vi "Run Optimization.vi"(8 "error in":errorcluster, 11 "Generic Optimization":refnum<class "Generic Optimization.lvclass">) -> (0 "error out":errorcluster, 3 "Generic Optimization out":refnum<class "Generic Optimization.lvclass">)   [LabVIEW 2018, in "Generic Optimization Actor.lvlib" / "Generic Optimization.lvclass"]
uses:
  Generic Optimization.lvclass
  C:/Users/Administrator/Desktop/LabVIEW EMS/EMS Generic Actor/EMS Generic/EMS Generic.lvclass
  Generic Optimization.lvclass/Generic Optimization.ctl
  EMS Generic Actor/EMS Generic/EMS Generic.lvclass
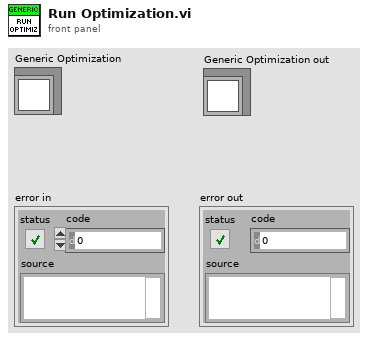
[diagram p1: front panel]
types:
  T1 = typedef "Generic Optimization Actor.lvlib/Generic Optimization.lvclass/Optimization Results Cluster.ctl" = cluster{"negated_net_battery_hold":dbl[][], " reactive_hold":dbl[][], " generatorpower_hold":dbl[][], " generatorreactive_hold":dbl[][], " PV_hold":dbl[][], "PCC_hold[0]":dbl[], " QCC_hold[0]":dbl[], " ES_VF_Controller":dbl[], " GEN_VF_Controller":dbl[], " voltage_hold":dbl[][], " SOC_hold":dbl[][], " Status":string}
  T2 = typedef "Generic Optimization Actor.lvlib/Generic Optimization.lvclass/Optimization Data Cluster.ctl" = cluster{"ES_BUS_ID":dbl[], "ES_VF_Controller":dbl[], "ES_Measurement_SOC":dbl[], "ES_Power_Rating":dbl[], "ES_Energy_Rating":dbl[], "ES_PowerFactor":dbl[], "ES_ChargeEffic":dbl[], "ES_DischargeEffic":dbl[], "ES_min_SOC":dbl[], "ES_max_SOC":dbl[], "GEN_BUS_ID":dbl[], "GEN_VF_Controller":dbl[], "GEN_Min_Power":dbl[], "GEN_Power_Rating":dbl[], "GEN_MaxPF_Lead":dbl[], "GEN_MaxPF_Lag":dbl[], "GEN_Marginal_Cost":dbl[][], "GEN_Marginal_Power":dbl[][], "GEN_Start_Cost":dbl[], "LOAD_BUS_ID":dbl[], "ForecastDataLongLoadP":dbl[][], "ForecastDataLongLoadQ":dbl[][], "PV_BUS_ID":dbl[], "PV_PowerRating_kVA":dbl[], "ForecastDataLongPV":dbl[][], "RealTimePrice":dbl[], "Forecast_dt":dbl, "Bus_Number":dbl[], "Bus_Voltage_Min":dbl[], "Bus_Voltage_Max":dbl[], "Bus_Voltage_Measured":dbl[], "Bus_Voltage_Nominal":dbl[], "From_Bus":dbl[], "To_Bus":dbl[], "Network_resistance":dbl[], "Network_reactance":dbl[], "Power_Flow_Limit":dbl[][], "Linear_PieceWise_PowerFLow":dbl[][], "Reactive_Flow_Limit":dbl[][], "Linear_PieceWise_ReactiveFLow":dbl[][], "PCC_min":dbl[], "PCC_max":dbl[], "QCC_min":dbl[], "QCC_max":dbl[], "Optimization_Type":i32, "Grid_State":i32}
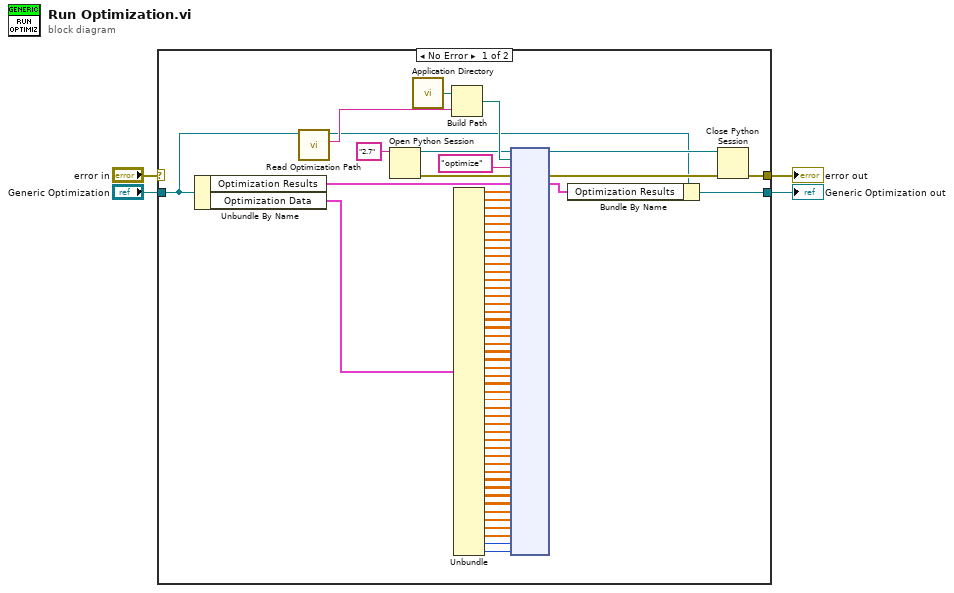
[diagram p0: block diagram]
diagram:
  n1 = case shown="No Error" "error in" {
    selector: "error in" -> [_ w68]
    tunnel: [w8 w68] -> w4
    tunnel: "Generic Optimization" -> [w7 w67]
    tunnel: [w14 w67] -> w1
    frame No Error {
      n2 = Unbundle By Name(w7) -> ("Optimization Results"=w63:T1, "Optimization Data"=w62:T2)
      n3 = call "Read Optimization Path.vi"("EMS Generic in"=w7) -> ("Optimization Relative Path"=w6:string, "EMS Generic out"=w5:refnum<class "Generic Optimization.lvclass">)  [unwired: 8 in, 1 out]
      n4 = Open Python Session(python version="2.7" ("Python version")) -> (session out=w12:refnum<k35>, error out=w11:errorcluster)  [unwired: 2 in]
      n5 = call <vilib>:"Application Directory.vi"() -> ("Application Directory"=w65:path)
      n6 = Build Path(base path=w65, name or relative path=w6) -> (appended path=w64:path)
      n7 = Unbundle(w62) -> ("ES_BUS_ID"=w61:dbl[], "ES_VF_Controller"=w60:dbl[], "ES_Measurement_SOC"=w59:dbl[], "ES_Power_Rating"=w58:dbl[], "ES_Energy_Rating"=w57:dbl[], "ES_PowerFactor"=w56:dbl[], "ES_ChargeEffic"=w55:dbl[], "ES_DischargeEffic"=w54:dbl[], "ES_min_SOC"=w53:dbl[], "ES_max_SOC"=w52:dbl[], "GEN_BUS_ID"=w51:dbl[], "GEN_VF_Controller"=w50:dbl[], "GEN_Min_Power"=w49:dbl[], "GEN_Power_Rating"=w48:dbl[], "GEN_MaxPF_Lead"=w47:dbl[], "GEN_MaxPF_Lag"=w46:dbl[], "GEN_Marginal_Cost"=w45:dbl[][], "GEN_Marginal_Power"=w44:dbl[][], "GEN_Start_Cost"=w43:dbl[], "LOAD_BUS_ID"=w42:dbl[], "ForecastDataLongLoadP"=w41:dbl[][], "ForecastDataLongLoadQ"=w40:dbl[][], "PV_BUS_ID"=w39:dbl[], "PV_PowerRating_kVA"=w38:dbl[], "ForecastDataLongPV"=w37:dbl[][], "RealTimePrice"=w36:dbl[], "Forecast_dt"=w35:dbl, "Bus_Number"=w34:dbl[], "Bus_Voltage_Min"=w33:dbl[], "Bus_Voltage_Max"=w32:dbl[], "Bus_Voltage_Measured"=w31:dbl[], "Bus_Voltage_Nominal"=w30:dbl[], "From_Bus"=w29:dbl[], "To_Bus"=w28:dbl[], "Network_resistance"=w27:dbl[], "Network_reactance"=w26:dbl[], "Power_Flow_Limit"=w25:dbl[][], "Linear_PieceWise_PowerFLow"=w24:dbl[][], "Reactive_Flow_Limit"=w23:dbl[][], "Linear_PieceWise_ReactiveFLow"=w22:dbl[][], "PCC_min"=w21:dbl[], "PCC_max"=w20:dbl[], "QCC_min"=w19:dbl[], "QCC_max"=w18:dbl[], "Optimization_Type"=w17:i32, "Grid_State"=w16:i32)
      n8 = node(w12, w64, "optimize" ("Function or Method Name"), w11, w63, w61, w60, w59, w58, w57, w56, w55, w54, w53, w52, w51, w50, w49, w48, w47, w46, w45, w44, w43, w42, w41, w40, w39, w38, w37, w36, w35, w34, w33, w32, w31, w30, w29, w28, w27, w26, w25, w24, w23, w22, w21, w20, w19, w18, w17, w16) -> (w10:refnum<k35>, w9:errorcluster, w15:T1)  [unwired: 46 in, 2 out]
      n9 = Bundle By Name(cluster=w5, "Optimization Results"=w15) -> (w14:refnum<class "Generic Optimization.lvclass">)
      n10 = Close Python Session(session in=w10, error in=w9) -> (11:w8:errorcluster)
    }
    frame Error {
    }
  }
  "error out" <- w4
  "Generic Optimization out" <- w1
